vi "CFU_4p2_TEAM072.vi"() -> ()   [LabVIEW 2016]
uses:
  <vilib>/express/express arith-compare/Formula/XNode/ExpressFormulaBlockNode.xnode
panel:
  in  "Names":string
  out "Kinetic Energy":dbl
  out "Moment of Interia, I (kg-m^2)":dbl
  in  "angular velocity, w (rad/s)":dbl
  in  "radius, r (m)":dbl
  in  "Mass, m (kg)":dbl
  in  "Inertial Constant k":dbl
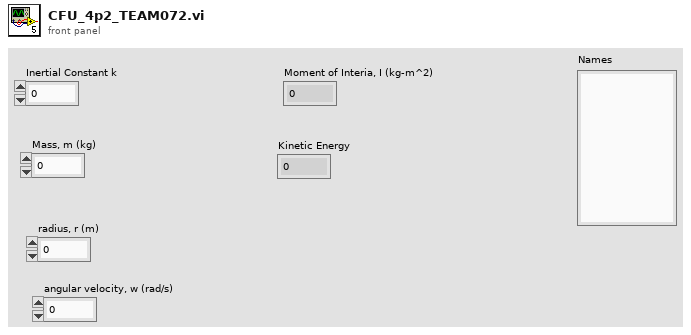
[diagram p1: front panel]
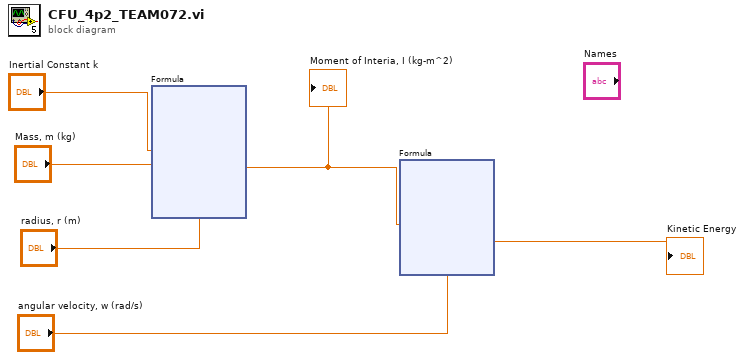
[diagram p0: block diagram]
diagram:
  n1 = xnode "Formula"("k"="Inertial Constant k", "m"="Mass, m (kg)", "r"="radius, r (m)") -> ("Result"=w3:dbl)  [unwired: 1 in, 1 out]
  "Moment of Interia, I (kg-m^2)" <- w3
  n2 = xnode "Formula"("I"=w3, "w"="angular velocity, w (rad/s)") -> ("Result"=→"Kinetic Energy":dbl)  [unwired: 1 in, 1 out]
